vi "Ejercicio_02_Verificar_info.vi"() -> ()   [LabVIEW 2020]
panel:
  out "Tarjeta confirmada":string
  in  "String":string
  in  "Table Control 2":string[][](table)
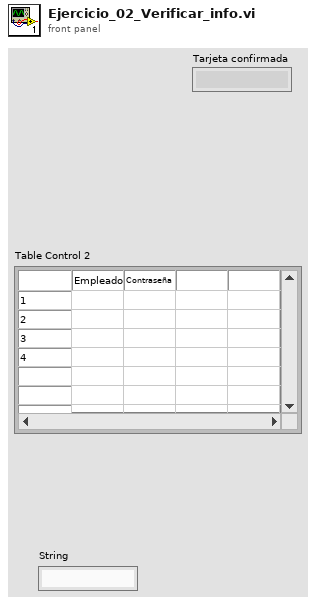
[diagram p1: front panel]
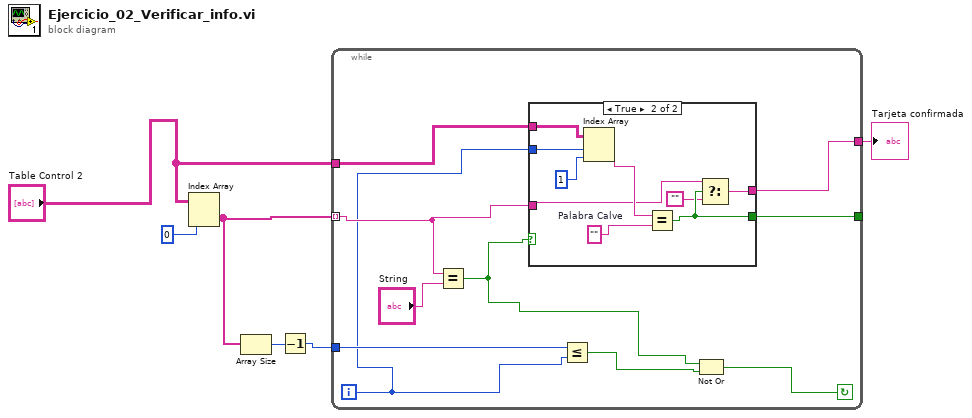
[diagram p0: block diagram]
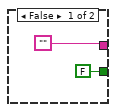
[diagram p2: hidden frame]
diagram:
  n1 = Index Array "Index Array"(array="Table Control 2", index (col)=0 ("disabled index (col)")) -> (element=w4:string[])  [unwired: 1 in]
  n2 = Array Size(array=w4) -> (size(s)=w6:i32)
  n3 = Decrement(x=w6) -> (x-1=w5:i32)
  n4 = while {
    tunnel: w5 -> [w14]
    tunnel: w4 -> [w13] mode=indexing
    tunnel: [w12] -> _
    tunnel: [w11] -> w1
    tunnel: "Table Control 2" -> [w10]
    i -> [w9]
    stop <- w16 continue-if-true
    n5 = Equal?(x=w13, y="String") -> (x = y?=w8:bool)
    n6 = case shown="True" w8 {
      tunnel: w10 -> [_ w22]
      tunnel: w13 -> [_ w25]
      tunnel: [FALSE w24] -> w12
      tunnel: ["" w23] -> w11
      tunnel: w9 -> [_ w21]
      frame False {
      }
      frame True {
        w19 = ""  # Palabra Calve
        n7 = Index Array(array=w22, index (row)=w21, index (col)=1) -> (element=w26:string)
        n8 = Equal?(x=w26, y=w19) -> (x = y?=w24:bool)
        n9 = Select(t=w25, s=w24, f="") -> (s? t:f=w23:string)
      }
    }
    n10 = Less Or Equal?(x=w14, y=w9) -> (x <= y?=w15:bool)
    n11 = Not Or(1:w15, 2:w8) -> (0:w16:bool)
  }
  "Tarjeta confirmada" <- w1
